vi "EMCCD_Stack.vi"(0 "VISA Stage":refnum<visa-resource-name>="COM5", 1 "EMCCD trigger port":tag="Dev1/port0/line0", 2 "Axis":T1[](array[typedef])=[enum."Z", enum."Y", enum."Z", enum."Z", enum."F", enum."V"], 3 "strPath":string="stringPathToOutput", 5 "Z Step Size (um)":dbl=0.2, 7 "Step Num":i32=1, 9 "Rep Num":i32=1, 11 "error in (no error)":errorcluster, 12 "Exposure time (s)":dbl=0.01, 13 "Offset":dbl, 14 "strPalette":string="C:\\Program Files\\Andor SOLIS\\GREY.PAL") -> (15 "error out":errorcluster)   [LabVIEW 2018]
uses:
  Drivers and controls/ASI/ASI_VIs/ASI Library/Shared_Serial/Axis Name.ctl
  <vilib>/Analysis/1siggen.llb/Ramp Pattern by Delta.vi
  <vilib>/Analysis/NI_AALBase.lvlib
panel:
  # "Default settings"
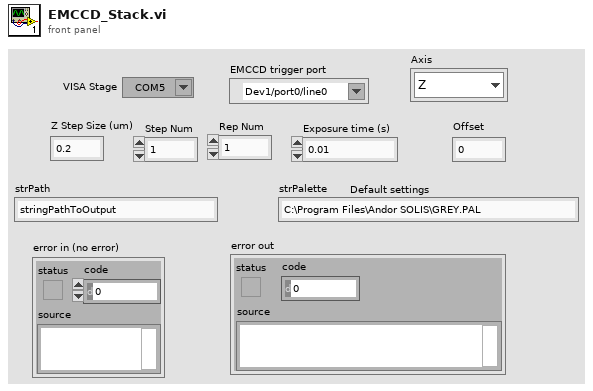
[diagram p1: front panel]
types:
  T1 = typedef "Axis Name.ctl" = enum8{"undefined", "A", "B", "C", "D", "E", "F", "G", "H", "I", "J", "K", "L", "M", "N", "O", "P", "Q", "R", "S", "T", "U", "V", "W", "X", "Y", "Z"}
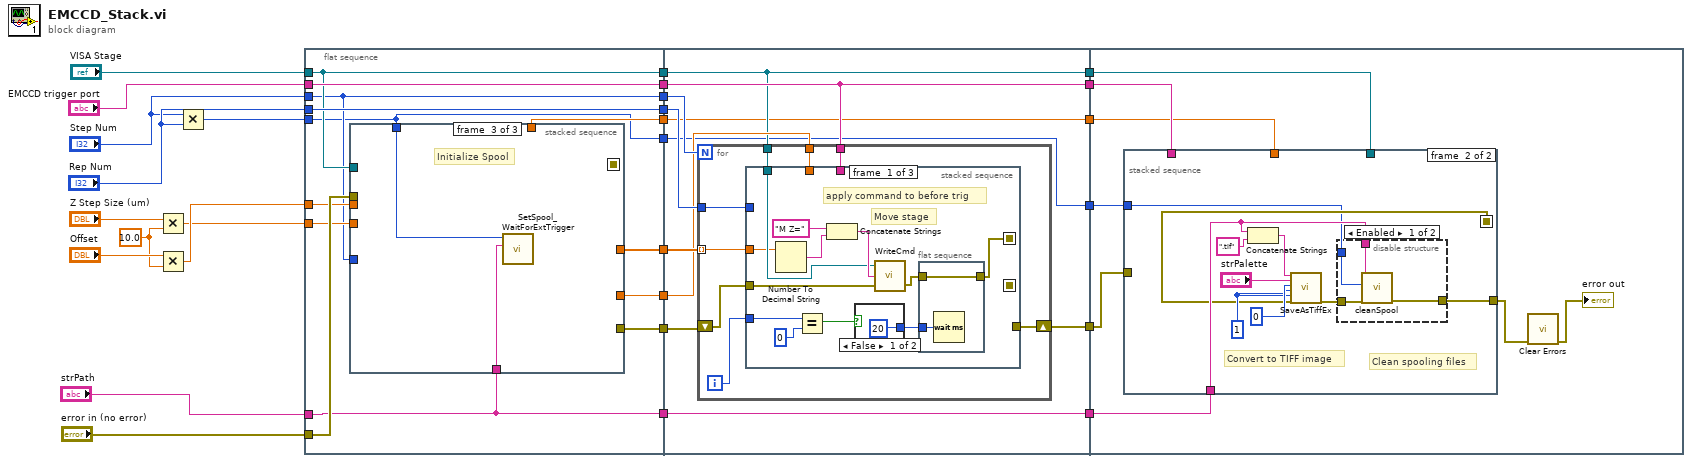
[diagram p0: block diagram]
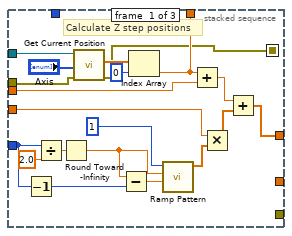
[diagram p2: hidden frame]
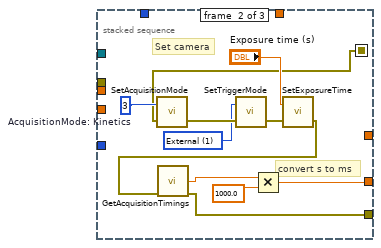
[diagram p3: hidden frame]
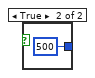
[diagram p4: hidden frame]
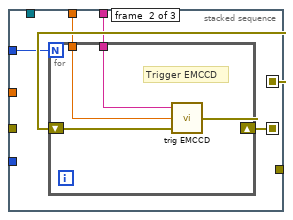
[diagram p5: hidden frame]
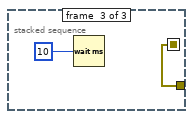
[diagram p6: hidden frame]
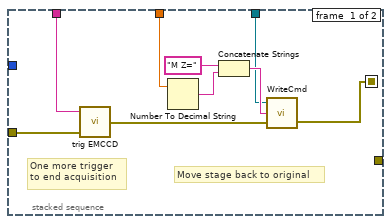
[diagram p7: hidden frame]
diagram:
  w11 = 10.0
  n1 = Multiply(x="Z Step Size (um)", y=w11) -> (x*y=w9:dbl)
  n2 = Multiply(x="Offset", y=w11) -> (x*y=w10:dbl)
  n3 = Multiply(x="Step Num", y="Rep Num") -> (x*y=w20:i32)
  n4 = flat-sequence {
    tunnel: "Rep Num" -> [w40]
    tunnel: "EMCCD trigger port" -> [w41]
    tunnel: "Step Num" -> [w35]
    tunnel: "error in (no error)" -> [w39]
    tunnel: [w35] -> w26
    tunnel: [w41] -> w25
    tunnel: [w40] -> w24
    tunnel: "strPath" -> [w33]
    tunnel: w20 -> [w29]
    tunnel: [w33] -> w18
    tunnel: "VISA Stage" -> [w38]
    tunnel: [w38] -> w15
    tunnel: w10 -> [w37]
    tunnel: w9 -> [w36]
    tunnel: [w34] -> w8
    tunnel: [w32] -> w7
    tunnel: [w31] -> w6
    tunnel: [w30] -> w3
    tunnel: [w29] -> w2
    tunnel: w26 -> [w84]
    tunnel: w25 -> [w81]
    tunnel: w24 -> [w83]
    tunnel: [w85] -> w23
    tunnel: [w82] -> w19
    tunnel: w18 -> [w82]
    tunnel: [w81] -> w17
    tunnel: w15 -> [w77]
    tunnel: w8 -> [w80]
    tunnel: w7 -> [w79]
    tunnel: w6 -> [w78]
    tunnel: [w77] -> w5
    tunnel: [w76] -> w4
    tunnel: w3 -> [w76]
    tunnel: w2 -> [w75]
    tunnel: [w75] -> w1
    tunnel: w23 -> [w127]
    tunnel: w19 -> [w128]
    tunnel: w17 -> [w126]
    tunnel: w5 -> [w125]
    tunnel: w4 -> [w124]
    tunnel: w1 -> [w123]
    frame #0 {
      n5 = stacked-sequence {
        seq-local: [w42 _ _] -> [_ w67 _]
        tunnel: w39 -> [w59 _ _]
        tunnel: w38 -> [w58 _ _]
        tunnel: w37 -> [w55 _ _]
        tunnel: [w54 _ _] -> w30
        tunnel: w36 -> [w52 _ _]
        tunnel: w35 -> [w45 _ _]
        tunnel: [w43 _ _] -> w34
        tunnel: w33 -> [_ _ w74]
        tunnel: w29 -> [_ _ w73]
        tunnel: [_ w63 _] -> w32
        tunnel: [_ w65 _] -> w31
        frame #0 {
          # "Calculate Z step positions"
          n6 = Decrement(x=w45) -> (x-1=w46:i32)
          n7 = Divide(x=w45, y=2.0) -> (x/y=w48:dbl)
          n8 = Round Toward -Infinity(1:w48) -> (0:w44:dbl)
          n9 = call "Get Current Position.vi"("error in (no error)"=w59, "Array of axes"="Axis", "VISA in"=w58) -> ("error out"=w42:errorcluster, "Array of positions [internal units]"=w56:dbl[])  [unwired: 6 in, 1 out]
          n10 = Subtract(x=w44, y=w46) -> (x-y=w47:dbl)
          n11 = Index Array(array=w56, index=0) -> (element=w54:dbl)
          n12 = call-poly <vilib>:"Ramp Pattern.vi"("start"=w47, "end"=w44, "delta"=1) -> ("Ramp Pattern"=w53:dbl[])  [unwired: 6 in, 2 out]
          n13 = Add(x=w54, y=w55) -> (x+y=w50:dbl)
          n14 = Multiply(x=w52, y=w53) -> (x*y=w51:dbl[])
          n15 = Add(x=w50, y=w51) -> (x+y=w43:dbl[])
        }
        frame #1 {
          w68 = u32 1 items=["Internal", "External"] ("Trigger")
          w69 = u16 3  # AcquisitionMode: Kinetics
          # "convert s to ms"
          # "Set camera"
          n16 = call <userlib>:"SetAcquisitionMode.vi"("error in (no error)"=w67, "mode"=w69) -> ("error out"=w71:errorcluster)  [unwired: 1 out]
          n17 = call <userlib>:"SetTriggerMode.vi"("error in (no error)"=w71, "mode"=w68) -> ("error out"=w72:errorcluster)  [unwired: 1 out]
          n18 = call <userlib>:"SetExposureTime.vi"("error in (no error)"=w72, "time"="Exposure time (s)") -> ("error out"=w66:errorcluster)  [unwired: 1 out]
          n19 = call <userlib>:"GetAcquisitionTimings.vi"("error in (no error)"=w66) -> ("kinetic"=w62:sgl, "error out"=w65:errorcluster)  [unwired: 10 in, 3 out]
          n20 = Multiply(x=w62, y=1000.0) -> (x*y=w63:dbl)
        }
        frame #2 {
          # "Initialize Spool"
          n21 = call "SetSpool_WaitForExtTrigger.vi"("path and name"=w74, "Kinetic Series"=w73) -> ()  [unwired: 10 in]
        }
      }
    }
    frame #1 {
      n22 = for {
        N: w84 -> [_]
        shift-right: [w90] -> w85
        shift-left: w78 -> [w91]
        tunnel: w81 -> [w93]
        tunnel: w83 -> [w92]
        tunnel: w79 -> [w89]
        tunnel: w77 -> [w88]
        tunnel: w80 -> [w86] mode=indexing
        i -> [w87]
        n23 = stacked-sequence {
          seq-local: [w95 _ _] -> [_ w114 _]
          seq-local: [_ w113 _] -> [_ _ w119]
          tunnel: w91 -> [w101 _ _]
          tunnel: w92 -> [_ w112 _]
          tunnel: w93 -> [_ w111 _]
          tunnel: [_ _ w119] -> w90
          tunnel: w89 -> [_ w110 _]
          tunnel: w88 -> [w100 _ _]
          tunnel: w87 -> [w97 _ _]
          tunnel: w86 -> [w94 _ _]
          frame #0 {
            # "Move stage"
            # "apply command to before trig"
            n24 = Number To Decimal String(number=w94) -> (decimal integer string=w104:string)  [unwired: 1 in]
            n25 = Equal?(x=w97, y=0) -> (x = y?=w99:bool)
            n26 = Concatenate Strings("M Z=", w104) -> (w103:string)
            n27 = case shown="False" w99 {
              tunnel: [20 500] -> w105
              frame False {
              }
              frame True {
              }
            }
            n28 = call "WriteCmd.vi"("error IO"=w101, "Command"=w103, "VISA resource name"=w100) -> ("error"=w96:errorcluster)  [unwired: 1 out]
            n29 = flat-sequence {
              tunnel: w105 -> [w107]
              tunnel: w96 -> [w106]
              tunnel: [w106] -> w95
              frame #0 {
                n30 = Wait (ms)(milliseconds to wait=w107) -> ()  [unwired: 1 out]
              }
            }
          }
          frame #1 {
            n31 = for {
              N: w112 -> [_]
              shift-right: [w117] -> w113
              shift-left: w114 -> [w118]
              tunnel: w111 -> [w116]
              tunnel: w110 -> [w115]
              # "Trigger EMCCD"
              n32 = call "trig EMCCD.vi"("error in (no error)"=w118, "camera time"=w115, "lines"=w116) -> ("error out"=w117:errorcluster)
            }
          }
          frame #2 {
            n33 = Wait (ms)(milliseconds to wait=10) -> ()  [unwired: 1 out]
          }
        }
      }
    }
    frame #2 {
      n34 = stacked-sequence {
        seq-local: [w131 _] -> [_ w139]
        tunnel: [_ w147] -> w122
        tunnel: w127 -> [w132 _]
        tunnel: w128 -> [_ w140]
        tunnel: w126 -> [w137 _]
        tunnel: w125 -> [w130 _]
        tunnel: w124 -> [w129 _]
        tunnel: w123 -> [_ w138]
        frame #0 {
          # "Move stage back to original"
          # "One more trigger\nto end acquisition"
          n35 = call "trig EMCCD.vi"("error in (no error)"=w132, "lines"=w137) -> ("error out"=w133:errorcluster)  [unwired: 1 in]
          n36 = Number To Decimal String(number=w129) -> (decimal integer string=w136:string)  [unwired: 1 in]
          n37 = Concatenate Strings("M Z=", w136) -> (w135:string)
          n38 = call "WriteCmd.vi"("error IO"=w133, "Command"=w135, "VISA resource name"=w130) -> ("error"=w131:errorcluster)  [unwired: 1 out]
        }
        frame #1 {
          w142 = 1
          # "Clean spooling files"
          # "Convert to TIFF image"
          n39 = Concatenate Strings(w140, ".tif") -> (w144:string)
          n40 = call <userlib>:"SaveAsTiffEx.vi"("path"=w144, "palette"="strPalette", "position"=0, "type"=w142, "mode"=w142, "error in (no error)"=w139) -> ("error out"=w146:errorcluster)  [unwired: 12 in, 1 out]
          n41 = disable-structure shown="Enabled" {
            disable-tunnel: [w151 w152] -> w147
            disable-tunnel: w146 -> [w150 w152]
            disable-tunnel: w140 -> [w149 _]
            disable-tunnel: w138 -> [w148 _]
            frame Enabled {
              n42 = call "cleanSpool.vi"("error in (no error)"=w150, "Total Img Num"=w148, "strPath"=w149) -> ("error out"=w151:errorcluster)  [unwired: 8 in]
            }
            frame Disabled {
            }
          }
        }
      }
      n43 = call <vilib>:"Clear Errors.vi"("error in (no error)"=w122) -> ("error out"=→"error out":errorcluster)  [unwired: 5 in, 1 out]
    }
  }
